vi "Take Line Image.vi"(0 "Gantry in":refnum<class "Gantry.lvclass">, 1 "Quality":enum16{"perfect", "high", "medium", "low"}(ring), 5 "Line Start":refnum<class "Vec3d.lvclass">, 9 "Line End":refnum<class "Vec3d.lvclass">, 11 "error in (no error)":errorcluster, 12 "Image Name":string="composite image", 13 "Slider Reference":refnum<vi>, 14 "Interrupt Reference":refnum<vi>) -> (4 "Gantry out":refnum<class "Gantry.lvclass">, 6 "Physical Image":T1, 15 "error out":errorcluster)   [LabVIEW 2024, in "Gantry.lvclass"]
uses:
  Gantry.lvclass
  Vec3d Class/Vec3d.lvclass
  Utils/Type Definitions/Physical Image.ctl
  <vilib>/vision/Image Controls.llb/IMAQ Image.ctl
  FlexWorktable/FlexWorktable.lvclass
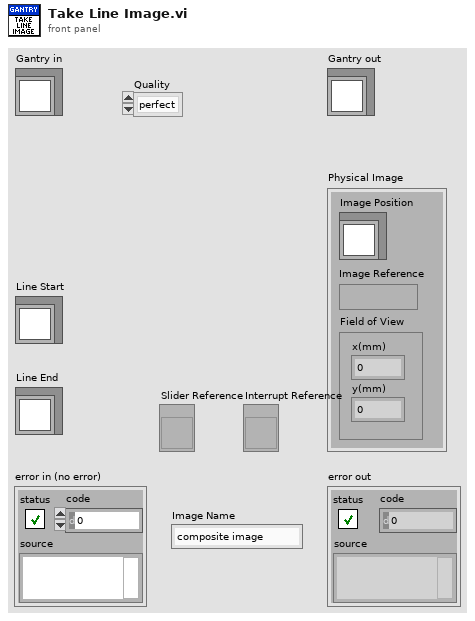
[diagram p1: front panel]
types:
  T1 = typedef "Physical Image.ctl" = cluster{"Image Position":refnum<class "Vec3d.lvclass">, "Image Reference":T2, "Field of View":cluster{"x(mm)":dbl, "y(mm)":dbl}}
  T2 = typedef "IMAQ Image.ctl" = refnum<image>
  T3 = typedef "FlexWorktable.lvclass/Camera State.ctl" = cluster{"Group":i32, "Open?":bool, "Driver":T4, "serial number":string, "Field of View":cluster{"x-mm":dbl, "y-mm":dbl}, "Rotation":T5, "Vertical Mirror":bool}
  T4 = typedef "Vision.lvlib/camera driver.ctl" = enum16{"none", "wmf", "imaqdx"}
  T5 = typedef "Camera Rotation.ctl" = enum16{"0", "90", "180", "270"}
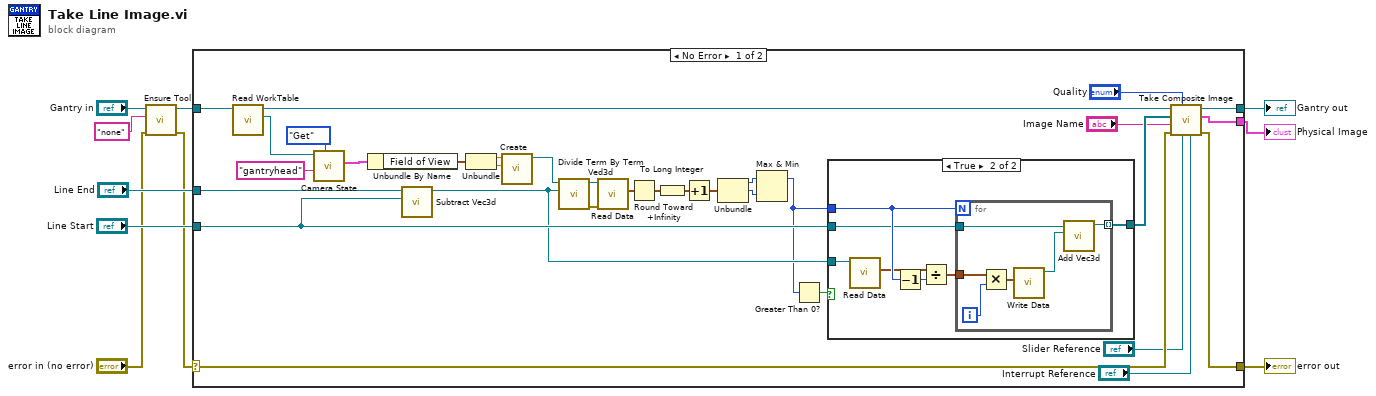
[diagram p0: block diagram]
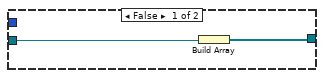
[diagram p2: hidden frame]
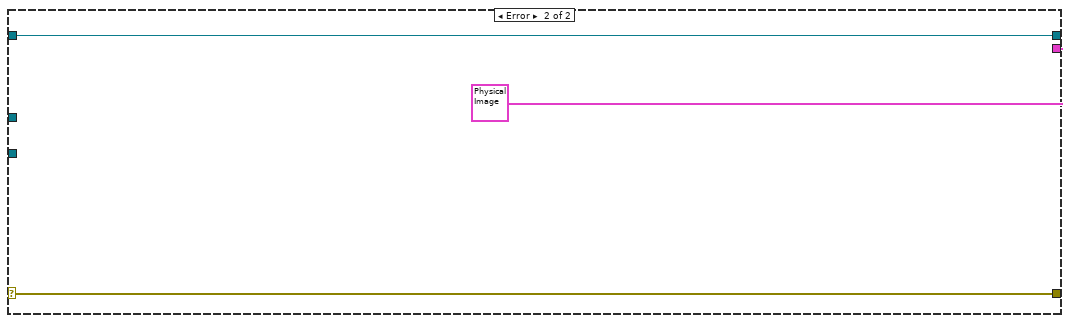
[diagram p3: hidden frame]
diagram:
  n1 = call "Ensure Tool.vi"("error in (no error)"="error in (no error)", "Tool Name"="none", "Gantry in"="Gantry in") -> ("error out"=w1:errorcluster, "Gantry out"=w4:refnum<class "Gantry.lvclass">)  [unwired: 7 in]
  n2 = case shown="No Error" w1 {
    selector: w1 -> [w34 w60]
    tunnel: [w33 w60] -> w6
    tunnel: [w35 w59] -> w8
    tunnel: w4 -> [w20 w59]
    tunnel: "Line End" -> [w31 _]
    tunnel: "Line Start" -> [w25 _]
    tunnel: [w32 T1 {"Image Position"=refnum, "Image Reference"=refnum, "Field of View"={"x(mm)"=0.0, "y(mm)"=0.0}} ("Physical Image")] -> w7
    frame No Error {
      n3 = call-dynamic "Read WorkTable.vi"("Gantry Class in"=w20) -> ("Worktable"=w19:refnum<class "FlexWorktable.lvclass">, "Gantry Class out"=w18:refnum<class "Gantry.lvclass">)  [unwired: 8 in, 1 out]
      n4 = call-dynamic "Camera State.vi"("Get/Set"=enum16{"Get", "Set"}."Get", "Camera Name"="gantryhead", "FlexWorktable in"=w19) -> ("State"=w16:T3)  [unwired: 6 in, 2 out]
      n5 = Unbundle By Name(w16) -> ("Field of View"=w40:cluster{"x-mm":dbl, "y-mm":dbl})
      n6 = call "Subtract Vec3d.vi"("Vec3d in 2"=w25, "Vec3d in 1"=w31) -> ("Vec3d Class out"=w24:refnum<class "Vec3d.lvclass">)  [unwired: 8 in, 1 out]
      n7 = Unbundle(w40) -> ("x-mm"=w42:dbl, "y-mm"=w41:dbl)
      n8 = call "Create.vi"("Y"=w41, "X"=w42) -> ("Vec3d Class out"=w36:refnum<class "Vec3d.lvclass">)  [unwired: 8 in, 1 out]
      n9 = call-dynamic "Divide Term By Term Ved3d.vi"("Vec3d in 2"=w24, "Vec3d in 1"=w36) -> ("error out"=w39:errorcluster, "Vec3d Class out"=w38:refnum<class "Vec3d.lvclass">)  [unwired: 8 in]
      n10 = call-dynamic "Read Data.vi"("error in (no error)"=w39, "Vec3d Class in"=w38) -> ("Data"=w37:cluster{"X":dbl, "Y":dbl, "Z":dbl})  [unwired: 7 in, 2 out]
      n11 = Round Toward +Infinity(x=w37) -> (ceil(x): smallest int >= x=w30:cluster{"X":dbl, "Y":dbl, "Z":dbl})
      n12 = To Long Integer(number=w30) -> (32bit integer=w29:cluster{"X":i32, "Y":i32, "Z":i32})
      n13 = Increment(x=w29) -> (x+1=w28:cluster{"X":i32, "Y":i32, "Z":i32})
      n14 = Unbundle(w28) -> ("X"=w27:i32, "Y"=w26:i32)  [unwired: 1 out]
      n15 = Max & Min(x=w27, y=w26) -> (max(x,y)=w22:i32)  [unwired: 1 out]
      n16 = Greater Than 0?(x=w22) -> (x > 0?=w23:bool)
      n17 = case shown="True" w23 {
        tunnel: [w43 w51] -> w21
        tunnel: w22 -> [_ w50]
        tunnel: w25 -> [w44 w48]
        tunnel: w24 -> [_ w47]
        frame False {
          n18 = Build Array(w44) -> (w43:refnum<class "Vec3d.lvclass">[])
        }
        frame True {
          n19 = call-dynamic "Read Data.vi"("Vec3d Class in"=w47) -> ("Data"=w46:cluster{"X":dbl, "Y":dbl, "Z":dbl})  [unwired: 8 in, 2 out]
          n20 = Decrement(x=w50) -> (x-1=w49:i32)
          n21 = Divide(x=w46, y=w49) -> (x/y=w45:cluster{"X":dbl, "Y":dbl, "Z":dbl})
          n22 = for {
            N: w50 -> [_]
            tunnel: [w57] -> w51 mode=indexing
            tunnel: w48 -> [w56]
            tunnel: w45 -> [w54]
            i -> [w53]
            n23 = Multiply(x=w54, y=w53) -> (x*y=w52:cluster{"X":dbl, "Y":dbl, "Z":dbl})
            n24 = call "Write Data.vi"("Data"=w52) -> ("Vec3d Class out"=w55:refnum<class "Vec3d.lvclass">)  [unwired: 9 in, 1 out]
            n25 = call-dynamic "Add Vec3d.vi"(10:"Vec3d Class in"=w55, 11:"Vec3d Class in"=w56) -> ("Vec3d Class out"=w57:refnum<class "Vec3d.lvclass">)  [unwired: 8 in, 1 out]
          }
        }
      }
      n26 = call "Take Composite Image.vi"("Interrupt Reference"="Interrupt Reference", "Slider Reference"="Slider Reference", "Quality"="Quality", "error in (no error)"=w34, "Image Name"="Image Name", "Points"=w21, "Gantry in"=w18) -> ("error out"=w33:errorcluster, "Physical Image"=w32:T1, "Gantry out"=w35:refnum<class "Gantry.lvclass">)  [unwired: 2 in]
    }
    frame Error {
    }
  }
  "error out" <- w6
  "Gantry out" <- w8
  "Physical Image" <- w7
